vi "UI SaveAs Config.vi"(8 "error in (no error)":errorcluster, 11 "UI_Left_Right in":refnum<class "Model_AMC.lvclass">) -> (0 "error out":errorcluster, 3 "UI_Left_Right out":refnum<class "Model_AMC.lvclass">)   [LabVIEW 2021, in "Model_AMC.lvclass"]
uses:
  Model_AMC.lvclass
  <userlib>/John_Lib/AbstractActorTemplate/AbstractActorTemplate/UIActorTop.lvclass
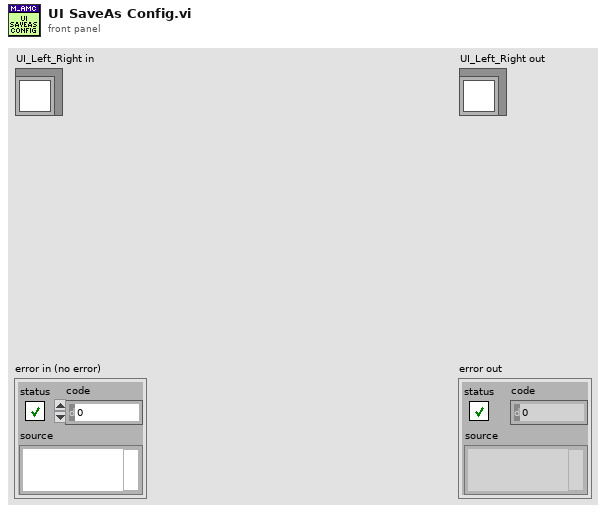
[diagram p1: front panel]
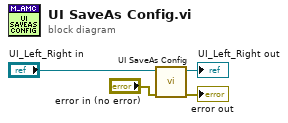
[diagram p0: block diagram]
diagram:
  n1 = call-parent "UI SaveAs Config.vi"("error in (no error)"="error in (no error)", "UIActorTop in"="UI_Left_Right in") -> ("error out"=→"error out":errorcluster, "UIActorTop out"=→"UI_Left_Right out":refnum<class "Model_AMC.lvclass">)  [unwired: 8 in]
